vi "open connection.vi"(8 "error in (no error)":errorcluster, 11 "tcp connection in":refnum<class "tcp connection.lvclass">) -> (0 "error out":errorcluster, 3 "tcp connection out":refnum<class "tcp connection.lvclass">)   [LabVIEW 2014, in "tcp connection.lvclass"]
uses:
  tcp connection.lvclass
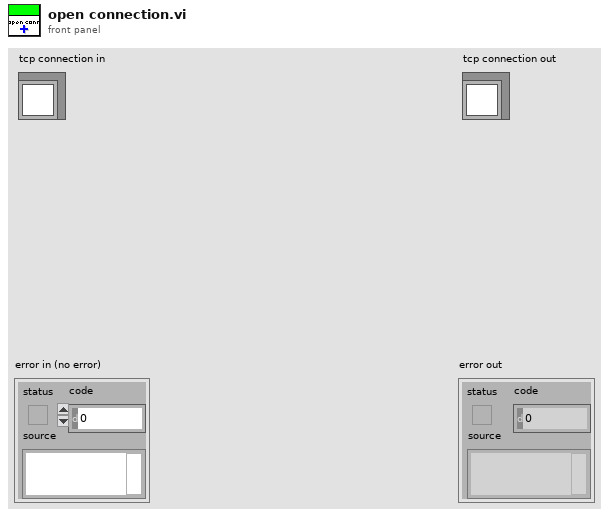
[diagram p1: front panel]
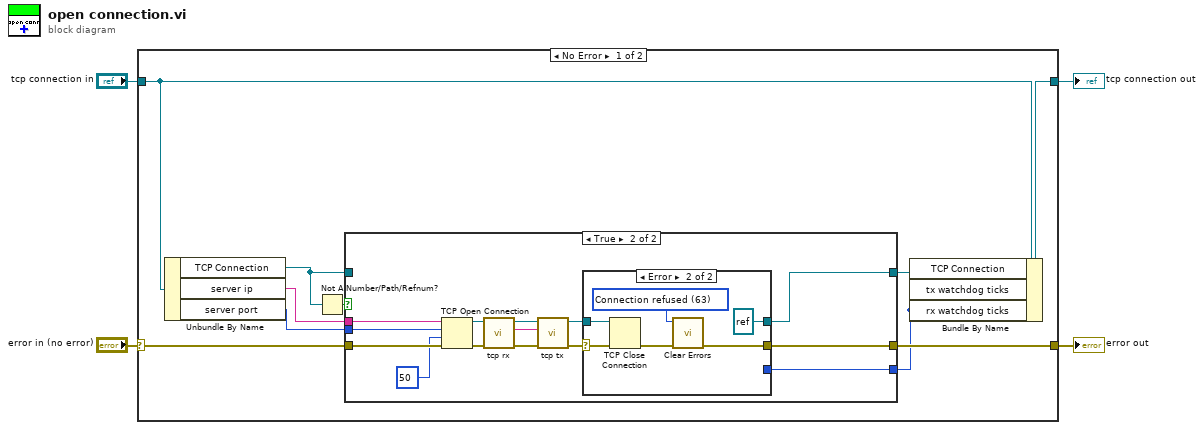
[diagram p0: block diagram]
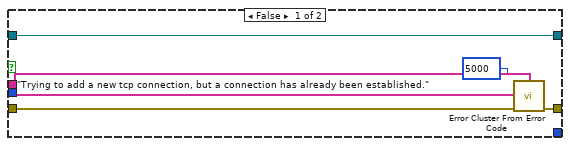
[diagram p2: hidden frame]
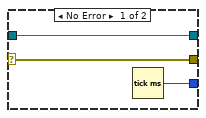
[diagram p3: hidden frame]
diagram:
  n1 = case shown="No Error" "error in (no error)" {
    selector: "error in (no error)" -> [w13 w44]
    tunnel: [w12 w44] -> w3
    tunnel: [w10 w43] -> w1
    tunnel: "tcp connection in" -> [w11 w43]
    frame No Error {
      n2 = Unbundle By Name(w11) -> ("TCP Connection"=w8:refnum<k5>, "server ip"=w7:string, "server port"=w6:i32)
      n3 = Not A Number/Path/Refnum?(number/path/refnum=w8) -> (NaN/Path/Refnum?=w14:bool)
      n4 = case shown="True" w14 {
        tunnel: w8 -> [w19 _]
        tunnel: [w19 w33] -> w9
        tunnel: [w17 w32] -> w12
        tunnel: w13 -> [w18 w31]
        tunnel: w7 -> [_ w30]
        tunnel: [_ w21] -> w5
        tunnel: w6 -> [_ w20]
        frame False {
          n5 = call <vilib>:"Error Cluster From Error Code.vi"("error in (no error)"=w18, "error message (\"\")"="Trying to add a new tcp connection, but a connection has already been established." ("error message (\"\")"), "error code (0)"=5000) -> ("error out"=w17:errorcluster)  [unwired: 6 in]
        }
        frame True {
          n6 = TCP Open Connection(address=w30, remote port or service name=w20, timeout ms (60000)=50, error in (no error)=w31) -> (connection ID=w28:refnum<k5>, error out=w27:errorcluster)  [unwired: 1 in]
          n7 = call "tcp rx.vi"("error in"=w27, "TCP Connection in"=w28) -> ("error out"=w25:errorcluster, "rx"=w24:string, "TCP Connection out"=w26:refnum<k5>)  [unwired: 6 in, 1 out]
          n8 = call "tcp tx.vi"("error in"=w25, "tx"=w24, "TCP Connection in"=w26) -> ("error out"=w22:errorcluster, "TCP Connection out"=w23:refnum<k5>)  [unwired: 7 in]
          n9 = case shown="Error" w22 {
            selector: w22 -> [w35 w40]
            tunnel: [w36 refnum<k5> refnum ("TCP Connection out")] -> w33
            tunnel: w23 -> [w36 w42]
            tunnel: [w35 w38] -> w32
            tunnel: [w34 _] -> w21
            frame No Error {
              n10 = Tick Count (ms)() -> (millisecond timer value=w34:u32)
            }
            frame Error {
              w37 = 63 items=["No Error", "Argument Error", "Memory Full", "Out of Zone", "End of File", "File Already Open", "Generic File IO Error", "File Not Found", "File Permission Error", "Disk Full", "Duplicate Path", "Too Many Files Open", "Not Enabled", "Resource File Not Found", "Cannot Add Resource", "Resource Not Found", "Image Not Found", "Image Memory Error", "Pen Does Not Exist", "Config Bad Type", "Config Token Not Found", "Config Parse Error", "Config Memory Error", "Bad External Code Format", "Bad External Code Offset", "External Code Not Present", "Null Window", "Destroy Window Mixup", "Null Menu", "Print Aborted", "Bad Print Record", "Print Driver Error", "Windows Error During Print", "Memory Error During Print", "Print Dialog Error", "Generic Print Error", "Invalid Device Refnum", "Device Not Found", "Device Parameter Error", "Device Unit Error", "Can't Open Device", "Device Call Aborted", "Generic Error", "Cancelled By User", "Object ID Too Low", "Object ID Too High", "Object Not In Heap", "Unknown Heap", "Bad DefProc ID", "DefProc Not In Table", "Message Out Of Range", "Null Method", "Unknown Message", "Manager Call Not Supported", "Bad address", "Connection In progress", "Connection timed out", "Connection is already in progress", "Network attribute not supported", "Network error", "Address in use", "System out of memory", "Connection aborted", "Connection refused", "Connection is not connected", "Connection is already connected", "Connection closed", "Initialize error (interapplication manager)", "Bad occurrence", "Wait on unbound occurrence handler", "Occurrence queue overflow", "Bad path", "Semaphore not signaled", "Unrecognized type (interapplication manager)"] ("1st Error to Convert")
              n11 = TCP Close Connection(connection ID=w42, error in (no error)=w40) -> (error out=w39:errorcluster)  [unwired: 1 in, 1 out]
              n12 = call <vilib>:"Clear Errors.vi"("error in (no error)"=w39, "specific error code to clear (0: all)"=w37) -> ("error out"=w38:errorcluster)  [unwired: 4 in, 1 out]
            }
          }
        }
      }
      n13 = Bundle By Name(cluster=w11, "TCP Connection"=w9, "tx watchdog ticks"=w5, "rx watchdog ticks"=w5) -> (w10:refnum<class "tcp connection.lvclass">)
    }
    frame Error {
    }
  }
  "error out" <- w3
  "tcp connection out" <- w1
